vi "ENPH354_A2Q3.vi"() -> ()   [LabVIEW 2020]
uses:
  <vilib>/Analysis/8numeric.llb/1D Numeric Integration.vi
  <vilib>/Analysis/NI_AALPro.lvlib
panel:
  out "Simulated Square Wave with Noise":dynamicdata(graph)=[{"t0"=timestamp(20.0939621925354 s since 1904-01-01), "dt"=0.0001, "Y"=array[1000 elements], "attributes"=variant("NI_ChannelName"=variant(string "Square with Uniform Noise"), "NI_ExpIsRelativeTime"=variant(bool TRUE), "NI_ExpStartTimeStamp"=variant(timestamp timestamp(3757653158.2169666 s since 1904-01-01)), "NI_ExpTimeStamp"=variant(timestamp timestamp(3757653178.310929 s since 1904-01-01)), "NI_ExpXDimension"=variant(string "t"))}]
  in  "stop":bool
  out "SUM vs. Duty Cycle":dbl(graph)
  # "ENPH354 Assignment 2 Q3"
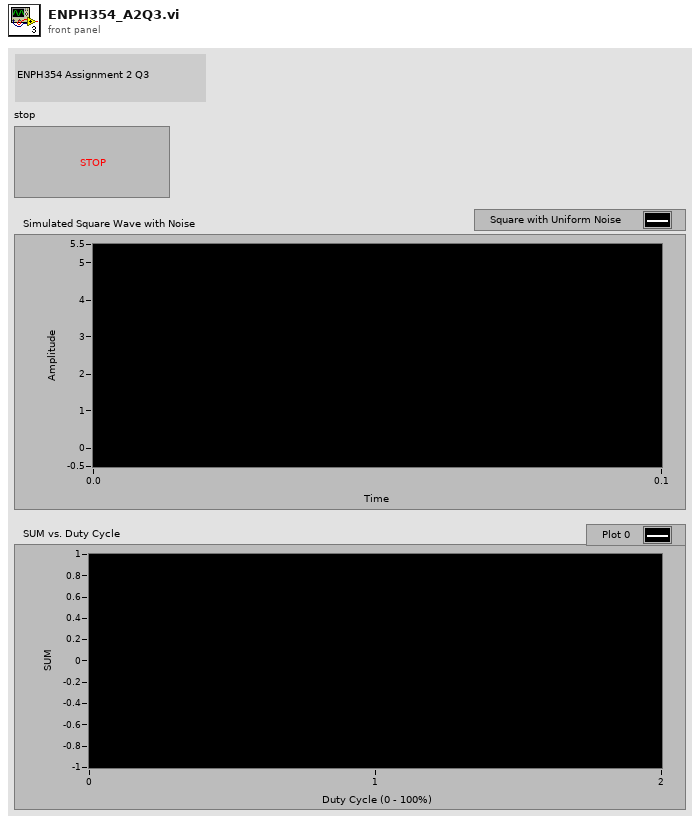
[diagram p1: front panel]
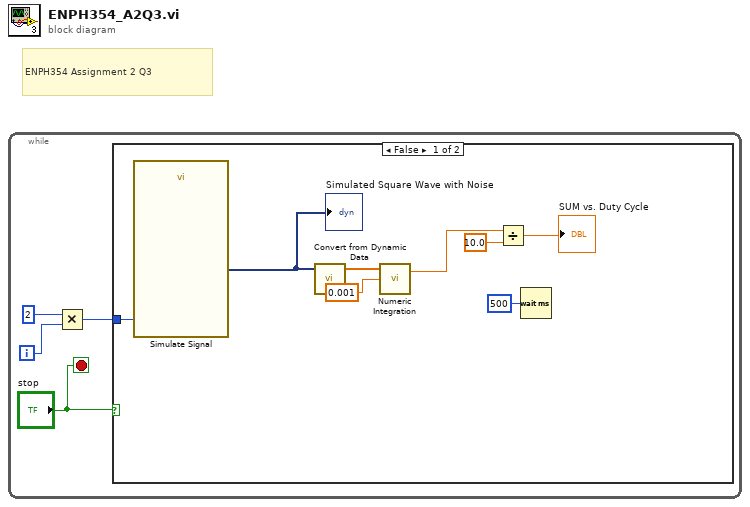
[diagram p0: block diagram]
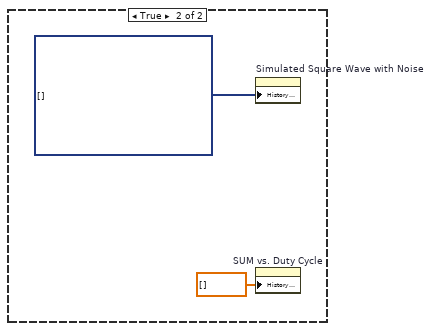
[diagram p2: hidden frame]
diagram:
  # "ENPH354 Assignment 2 Q3"
  n1 = while {
    i -> [w1]
    stop <- "stop" stop-if-true
    n2 = Multiply(x=2, y=w1) -> (x*y=w3:i32)
    n3 = case shown="False" "stop" {
      tunnel: w3 -> [w6 _]
      frame False {
        n4 = call "Simulate Signal"("Duty Cycle (%)"=w6) -> ("Square with Uniform Noise"=w8:dynamicdata)  [unwired: 13 in, 1 out]
        "Simulated Square Wave with Noise" <- w8
        n5 = call "Convert from Dynamic Data"("Dynamic Data Type"=w8) -> ("Array"=w11:dbl[])  [unwired: 3 in]
        n6 = call-poly <vilib>:"Numeric Integration.vi"("dt"=0.001, "Input Array"=w11) -> ("result"=w9:dbl)  [unwired: 1 in, 1 out]
        n7 = Divide(x=w9, y=10.0) -> (x/y=→"SUM vs. Duty Cycle":dbl)
        n8 = Wait (ms)(milliseconds to wait=u32 500) -> ()  [unwired: 1 out]
      }
      frame True {
        n9 = property on="Simulated Square Wave with Noise" class="WFChart (strict)"("History Data"=dynamicdata[] []) -> ()  [unwired: 2 in, 2 out]
        n10 = property on="SUM vs. Duty Cycle" class="WFChart (strict)"("History Data"=dbl[] []) -> ()  [unwired: 2 in, 2 out]
      }
    }
  }
